vi "Spline Interpolation 1D.vi"(4 "final boundary":T1, 6 "initial boundary":T1, 9 "xi":dbl[](array[numeric]) format="%_6g", 10 "X":dbl[](array[numeric]), 11 "Y":dbl[](array[numeric])) -> (0 "error":i32, 1 "piecewise polynomial":T2 {"x locations" format="%.4g"; "coefficients" format="%.4g"}, 3 "yi":dbl[](array[numeric]) format="%_6g")   [LabVIEW 2010, in "NI_Gmath.lvlib"]
doc: "Performs one-dimensional interpolation using the spline interpolation method based on the lookup table defined by <B>X</B> and <B>Y</B>."
uses:
  NI_Gmath.lvlib
  in_piecewise interp poly control.ctl
  Solve Linear Equations (single right hand).vi
  NI_AALPro.lvlib
panel:
  # "Spline Interpolation 1D"
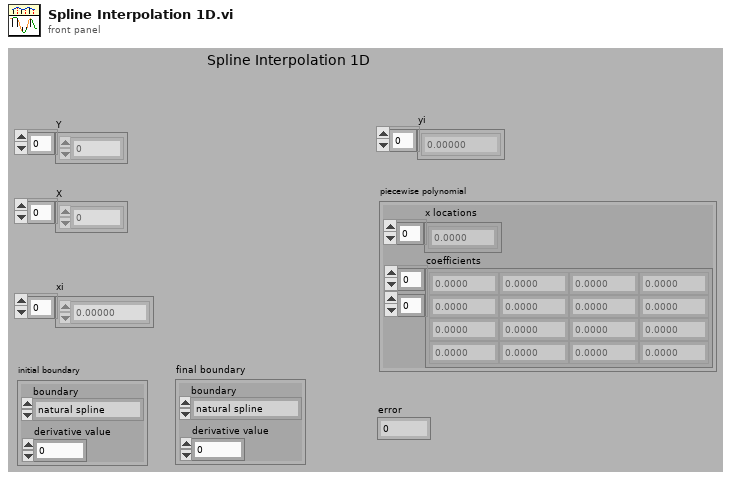
[diagram p1: front panel]
types:
  T1 = cluster{"boundary":enum16{"natural spline", "not-a-knot", "1st derivative", "2nd derivative"}, "derivative value":dbl}
  T2 = typedef "NI_Gmath.lvlib/in_piecewise interp poly control.ctl" = cluster{"x locations":dbl[], "coefficients":dbl[][]}
  T3 = typedef "NI_Matrix.lvlib/RealMatrix.ctl" = dbl[][]
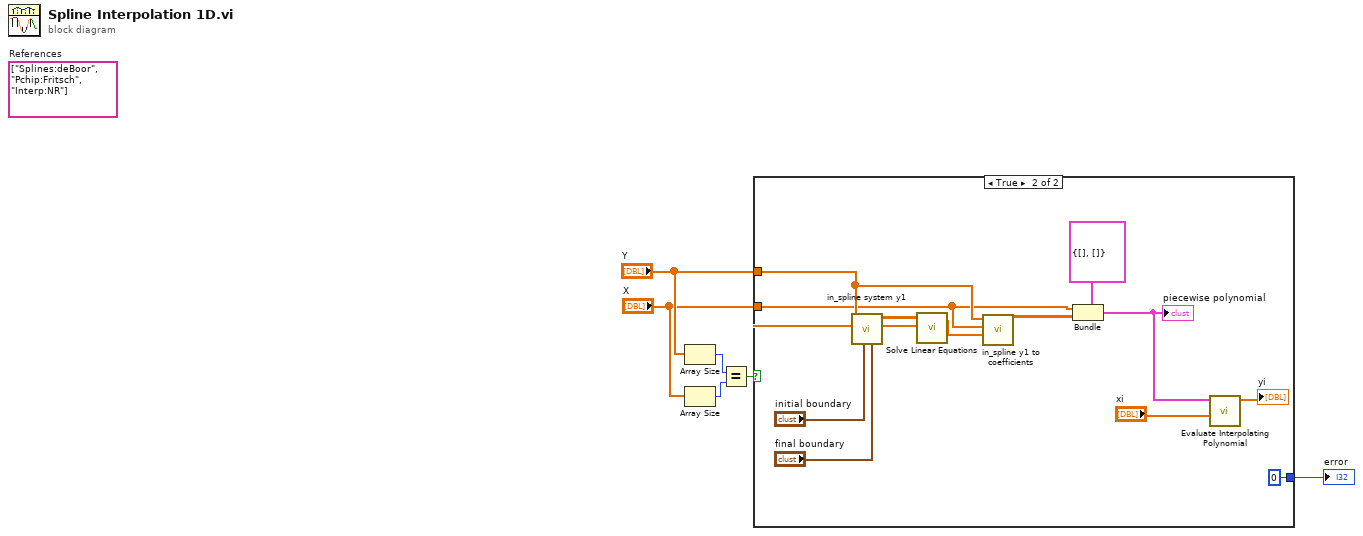
[diagram p0: block diagram]
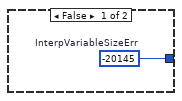
[diagram p2: hidden frame]
diagram:
  (unwired) string[] ["Splines:deBoor", "Pchip:Fritsch", "Interp:NR"]  # References
  n1 = Array Size(array="Y") -> (size(s)=w6:i32)
  n2 = Array Size(array="X") -> (size(s)=w5:i32)
  n3 = Equal?(x=w6, y=w5) -> (x = y?=w2:bool)
  n4 = case shown="True" w2 {
    tunnel: "Y" -> [_ w10]
    tunnel: "X" -> [_ w9]
    tunnel: [w7 0 ("error")] -> w1
    frame False {
      w7 = -20145  # InterpVariableSizeErr
    }
    frame True {
      n5 = call "in_spline system y1.vi"("final boundary"="final boundary", "initial boundary"="initial boundary", "X"=w9, "Y"=w10) -> ("b"=w19:dbl[], "A"=w20:T3)  [unwired: 6 in]
      n6 = call-poly "Solve Linear Equations.vi"("Known Vector"=w19, "Input Matrix"=w20) -> ("Solution Vector"=w18:dbl[])  [unwired: 1 in, 1 out]
      n7 = call "in_spline y1 to coefficients.vi"("Y1"=w18, "X"=w9, "Y"=w10) -> ("coefficients"=w17:dbl[][])  [unwired: 8 in]
      n8 = Bundle(cluster=T2 {"x locations"=[], "coefficients"=[]} ("piecewise polynomial"), "x locations"=w9, "coefficients"=w17) -> (w16:T2)
      "piecewise polynomial" <- w16
      n9 = call "Evaluate Interpolating Polynomial.vi"("xi"="xi", "piecewise polynomial"=w16) -> ("yi"=→"yi":dbl[])  [unwired: 8 in, 1 out]
    }
  }
  "error" <- w1
